vi "Close.vi"(8 "error in (no error)":errorcluster, 11 "RS232 in":refnum<class "RS-xxx.lvclass">) -> (0 "error out":errorcluster, 3 "RS232 out":refnum<class "RS-xxx.lvclass">)   [LabVIEW 2019, in "Protocols.lvlib" / "RS-xxx.lvclass"]
uses:
  RS-xxx.lvclass
  RS-xxx.lvclass/RS-xxx.ctl
  Data Access/Read Port Ref.vi
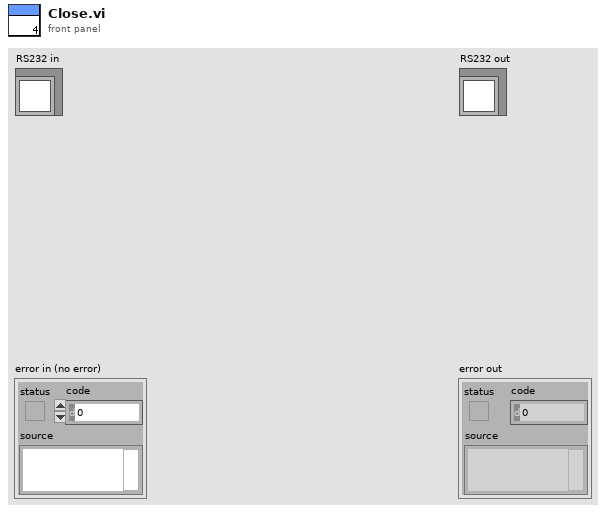
[diagram p1: front panel]
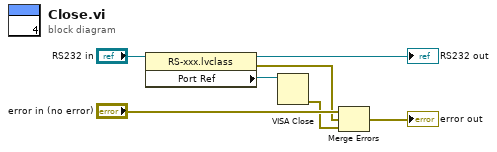
[diagram p0: block diagram]
diagram:
  n1 = property class="RS-xxx.lvclass"(reference="RS232 in") -> (reference out=→"RS232 out":refnum<class "RS-xxx.lvclass">, error out=w1:errorcluster, "Port Ref"=w6:refnum<visa-resource-name>)  [unwired: 1 in]
  n2 = VISA Close(VISA resource name=w6) -> (error out=w2:errorcluster)  [unwired: 1 in]
  n3 = Merge Errors("error in (no error)", w1, w2) -> (→"error out":errorcluster)
